vi "PID tester gyro.vi"   [LabVIEW 2016]
uses:
  <vilib>/NXT/Block Support/NXT_ButtonSelector.ctl
  <vilib>/NXT/Dual Mode Library/Waits/Wait_Btn.vi
types:
  T1 = typedef "NXT_ButtonSelector.ctl" = u16
  T2 = typedef "LVHSConnector.ctl" = refnum<class "BrickReference.lvclass">
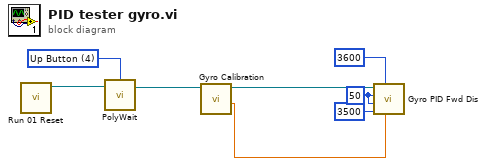
[diagram p0: block diagram]
diagram:
  w3 = T1 4 items=["Enter button"=3, "Left button"=2, "Right button"=1, "Up Button"=4, "Down Button"=5] ("Button (Enter button)")
  w5 = 50 ("Max. speed")
  n1 = call "Run 01 Reset.vi"() -> ("NXT/EV3 out"=w1:T2)  [unwired: 11 in]
  n2 = call-poly <vilib>:"PolyWait.vi"("NXT/EV3"=w1, "Button (Enter button)"=w3) -> ("NXT/EV3"=w2:T2)  [unwired: 2 in]
  n3 = call "Gyro Calibration.vi"("NXT/EV3"=w2) -> ("Degrees"=w7:sgl, "NXT/EV3"=w8:T2)  [unwired: 6 in, 1 out]
  n4 = call "Gyro PID Fwd Dis.vi"("Target angle"=w7, "Threshold to stop"=3600, "Threshold to slow"=3500, "Min. speed"=w5, "Max. speed"=w5, "EV3 in"=w8) -> ()  [unwired: 5 in, 1 out]
